vi "全局非断电保持变量.vi"() -> ()   [LabVIEW 2016, in "main.lvlib"]
uses:
  main.lvlib
panel:
  in  "EXO2实时数据":T1={"时间"=timestamp(0 s since 1904-01-01), "测量模式"="水样测试", "数据类型"="N", "数据标识"="N", "湖面水深"=0.0, "缆绳下放长度"=0.0, "层数"=0, "Temp"=0.0, "SpCond"=0.0, "Cond"=0.0, "Sal"=0.0, "TDS"=0.0, "pH"=0.0, "pHmV"=0.0, "ORP"=0.0, "DO"=0.0, "DO%"=0.0, "Turb"=0.0, "Chla"=0.0, "Depth"=0.0}
  in  "BBE实时数据":T2={"时间"=timestamp(0 s since 1904-01-01), "测量模式"="水样测试", "数据类型"="N", "数据标识"="N", "湖面水深"=0.0, "缆绳下放长度"=0.0, "层数"=0, "Temp"=0.0, "DO"=0.0, "DO%"=0.0, "GreenAlgae"=0.0, "BlueGreen"=0.0, "Diatoms"=0.0, "Cryptophyta"=0.0, "Transmission"=0.0, "Depth"=0.0}
  in  "BBE仪器测试数据":T2[](array[typedef])
  in  "EXO2仪器测试数据":T1[](array[typedef])
  out "运行状态":bool
  out "位置变化值":dbl
  out "剖面路径":dbl[](array[numeric])
  out "日志":string
  in  "监测数据":string[][](table)
  out "声纳通讯":bool
  out "仪器通讯":bool
  out "IO通讯":bool
  out "仪器电源":bool
  out "剖面下降":bool
  out "剖面上升":bool
  in  "仪器位置":dbl format="%#_6f m"
  out "湖面水深":dbl format="%#_6f m"
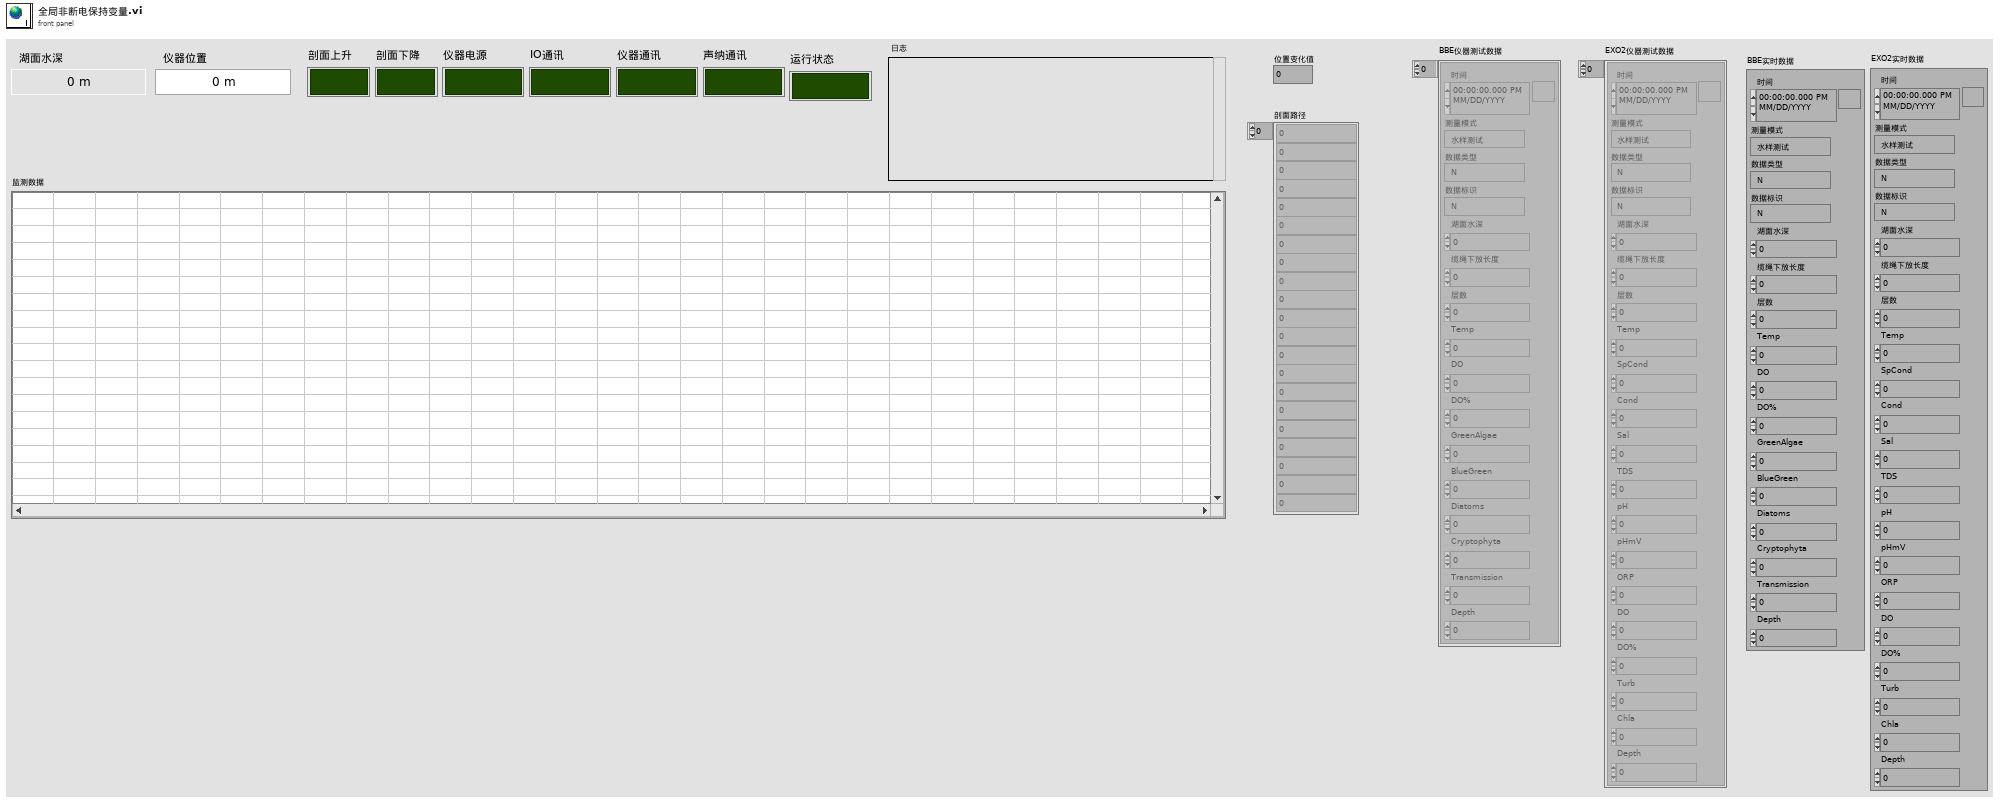
[diagram p1: front panel]
types:
  T1 = typedef "剖面数据_EXO2.ctl" = cluster{"时间":timestamp, "测量模式":string, "数据类型":string, "数据标识":string, "湖面水深":sgl, "缆绳下放长度":sgl, "层数":u16, "Temp":sgl, "SpCond":sgl, "Cond":sgl, "Sal":sgl, "TDS":sgl, "pH":sgl, "pHmV":sgl, "ORP":sgl, "DO":sgl, "DO%":sgl, "Turb":sgl, "Chla":sgl, "Depth":sgl}
  T2 = typedef "剖面数据_bbe_NAQDO.ctl" = cluster{"时间":timestamp, "测量模式":string, "数据类型":string, "数据标识":string, "湖面水深":sgl, "缆绳下放长度":sgl, "层数":u16, "Temp":sgl, "DO":sgl, "DO%":sgl, "GreenAlgae":sgl, "BlueGreen":sgl, "Diatoms":sgl, "Cryptophyta":sgl, "Transmission":sgl, "Depth":sgl}
diagram:
